vi "DAQ.vi"() -> (1 "Amperage across shunt":dbl, 2 "Light Resistance":dbl, 3 "Temperature in Celsius":dbl)   [LabVIEW 2011]
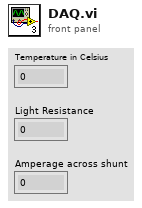
[diagram p1: front panel]
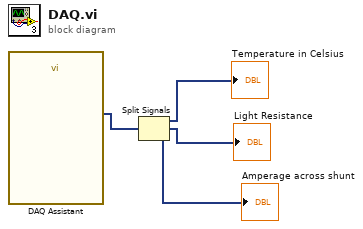
[diagram p0: block diagram]
diagram:
  n1 = call "DAQ Assistant"() -> ("data"=w1:dynamicdata)  [unwired: 17 in, 2 out]
  n2 = Split Signals(w1) -> (→"Temperature in Celsius":dynamicdata, →"Light Resistance":dynamicdata, →"Amperage across shunt":dynamicdata)  [unwired: 3 in]
